vi "CameraStatusTempGood.vi"(8 "error in (no error)":errorcluster, 9 "camera":u16, 10 "block":u32, 11 "sample":u32) -> (0 "error out":errorcluster, 3 "temp":bool)   [LabVIEW 2015, in "ESLSCDLL.lvlib"]
uses:
  ESLSCDLL.lvlib
  Globals.vi
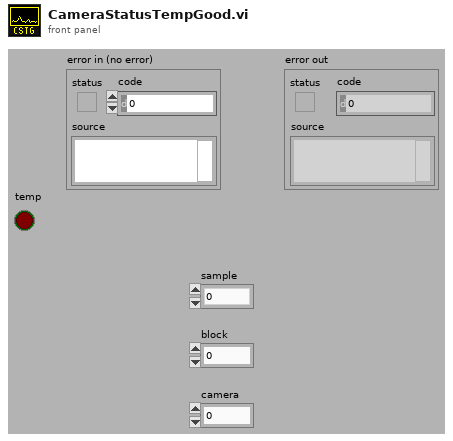
[diagram p1: front panel]
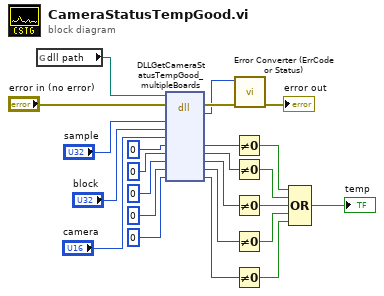
[diagram p0: block diagram]
diagram:
  n1 = global read "Globals.vi" "dll path"() -> (w1:path)
  n2 = dll-call lib="C:/ENTW/PCIE/LV64/board.vis/ESLSCDLL.dll" fn="DLLGetCameraStatusTempGood_multipleBoards" ("lwlscdll.dll:DLLWriteLongS0")(path in=w1, error in="error in (no error)", "sample"="sample", "block"="block", "camera_pos"="camera", "tempGood1"=u8 0, "tempGood2"=u8 0, "tempGood3"=u8 0, "tempGood4"=u8 0, "tempGood5"=u8 0) -> (error out=w22:errorcluster, "es_status_codes"=w21:i32, "tempGood1"=w8:u8, "tempGood2"=w9:u8, "tempGood3"=w10:u8, "tempGood4"=w11:u8, "tempGood5"=w12:u8)  [unwired: 4 in, 1 out]
  n3 = Not Equal To 0?(x=w8) -> (x != 0?=w7:bool)
  n4 = Not Equal To 0?(x=w9) -> (x != 0?=w6:bool)
  n5 = Not Equal To 0?(x=w10) -> (x != 0?=w5:bool)
  n6 = Not Equal To 0?(x=w11) -> (x != 0?=w4:bool)
  n7 = Not Equal To 0?(x=w12) -> (x != 0?=w3:bool)
  n8 = call "Error Converter (ErrCode or Status).vi"("error in (no error)"=w22, "error code"=w21) -> ("error out"=→"error out":errorcluster)  [unwired: 9 in]
  n9 = Compound Arithmetic op=OR(w7, w6, w5, w4, w3) -> (→"temp":bool)
